vi "AKD Close.vi"(0 "connection ID":refnum<k5>, 11 "error in":errorcluster) -> (15 "error out":errorcluster)   [LabVIEW 2024]
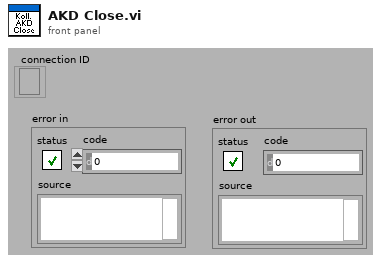
[diagram p1: front panel]
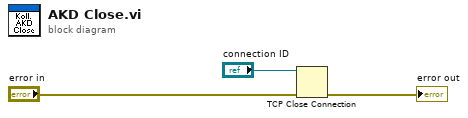
[diagram p0: block diagram]
diagram:
  n1 = TCP Close Connection(connection ID="connection ID", error in (no error)="error in") -> (error out=→"error out":errorcluster)  [unwired: 1 in, 1 out]
